vi "AssertControlDisable_Tests.vi"(11 "error in":errorcluster) -> (15 "error out":errorcluster)   [LabVIEW 2016, in "DronaTest.lvlib"]
uses:
  DronaTest.lvlib
  APIs/Stimulus/ControlValue/ValueSignalByPathString.vi
  APIs/Assert/AssertControlProperty/AssertControlDisable/AssertDisabled.vi
  APIs/Assert/AssertControlProperty/AssertControlDisable/AssertDisabledAndGrayedOut.vi
  APIs/Assert/AssertControlProperty/AssertControlDisable/AssertEnabled.vi
  <vilib>/addons/_JKI Toolkits/Caraya/classes/Test/Test.lvclass
  Drona.lvlib
  APIs/Stimulus/ControlValue/ControlValue.lvlib
  <vilib>/addons/_JKI Toolkits/Caraya/classes/Assert/Assert.lvclass
  APIs/Assert/AssertControlProperty/AssertControlDisable/AssertControlDisable.lvlib
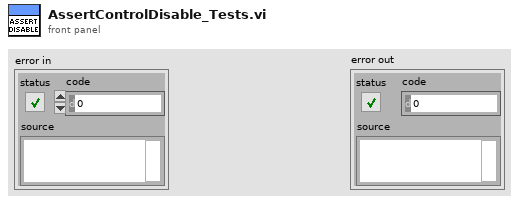
[diagram p1: front panel]
types:
  T1 = enum8{"Enabled", "Disabled", "Disabled and Grayed Out"}
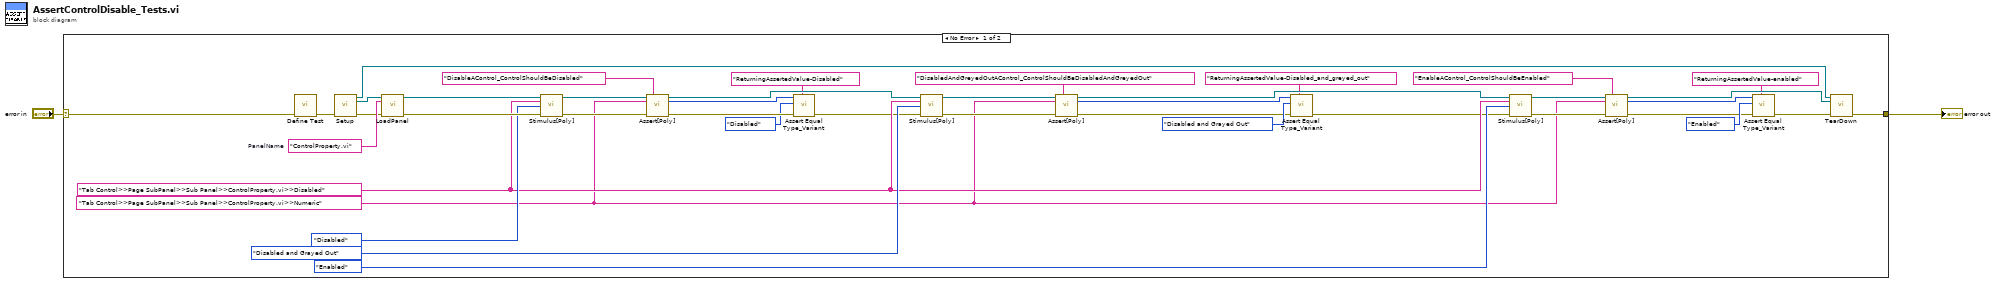
[diagram p0: block diagram]
diagram:
  n1 = case shown="No Error" "error in" {
    selector: "error in" -> [w43 w44]
    tunnel: [w20 w44] -> w1
    frame No Error {
      w24 = "Tab Control>>Page SubPanel>>Sub Panel>>ControlProperty.vi>>Numeric" ("Control Path")
      w25 = "Tab Control>>Page SubPanel>>Sub Panel>>ControlProperty.vi>>Disabled" ("Control Path")
      w42 = "ControlProperty.vi"  # PanelName
      n2 = call <vilib>:"Define Test.vi"("error in (no error)"=w43) -> ("error out"=w21:errorcluster)  [unwired: 9 in, 1 out]
      n3 = call "Setup.vi"("error in"=w21) -> ("Application Ref"=w18:refnum<vi>, "VI out"=w22:refnum<vi>, "error out"=w23:errorcluster)  [unwired: 12 in]
      n4 = call "LoadPanel.vi"("VI in"=w22, "Item Name"=w42, "error in"=w23) -> ("VI out"=w40:refnum<vi>, "error out"=w37:errorcluster)  [unwired: 11 in]
      n5 = call-poly "Stimulus[Poly].vi"("VI Reference In"=w40, "Control Path"=w25, "Value (Signaling)"=T1."Disabled" ("Disabled"), "error in"=w37) -> ("VI Reference Out"=w39:refnum<vi>, "error out"=w41:errorcluster)  [unwired: 10 in]
      n6 = call-poly "Assert[Poly].vi"("VI Reference In"=w39, "Test Label"="DisableAControl_ControlShouldBeDisabled" ("string"), "Control Path"=w24, "Error In"=w41) -> ("VI Reference Out"=w31:refnum<vi>, "Asserted Value"=w15:T1, "Error Out"=w17:errorcluster)  [unwired: 9 in]
      n7 = call <vilib>:"Assert Equal Type_Variant.vi"("Label"="ReturningAssertedValue-Disabled", "error in (no error)"=w17, "Y"=T1."Disabled" ("Asserted Value"), "X"=w15) -> ("error out"=w16:errorcluster)  [unwired: 6 in, 1 out]
      n8 = call-poly "Stimulus[Poly].vi"("VI Reference In"=w31, "Control Path"=w25, "Value (Signaling)"=T1."Disabled and Grayed Out" ("Disabled"), "error in"=w16) -> ("VI Reference Out"=w33:refnum<vi>, "error out"=w32:errorcluster)  [unwired: 10 in]
      n9 = call-poly "Assert[Poly].vi"("VI Reference In"=w33, "Test Label"="DisabledAndGreyedOutAControl_ControlShouldBeDisabledAndGreyedOut" ("string"), "Control Path"=w24, "Error In"=w32) -> ("VI Reference Out"=w27:refnum<vi>, "Asserted Value"=w8:T1, "Error Out"=w10:errorcluster)  [unwired: 9 in]
      n10 = call <vilib>:"Assert Equal Type_Variant.vi"("Label"="ReturningAssertedValue-Disabled_and_greyed_out", "error in (no error)"=w10, "Y"=T1."Disabled and Grayed Out" ("Asserted Value"), "X"=w8) -> ("error out"=w9:errorcluster)  [unwired: 6 in, 1 out]
      n11 = call-poly "Stimulus[Poly].vi"("VI Reference In"=w27, "Control Path"=w25, "Value (Signaling)"=T1."Enabled" ("Disabled"), "error in"=w9) -> ("VI Reference Out"=w29:refnum<vi>, "error out"=w30:errorcluster)  [unwired: 10 in]
      n12 = call-poly "Assert[Poly].vi"("VI Reference In"=w29, "Test Label"="EnableAControl_ControlShouldBeEnabled" ("string"), "Control Path"=w24, "Error In"=w30) -> ("VI Reference Out"=w19:refnum<vi>, "Asserted Value"=w3:T1, "Error Out"=w5:errorcluster)  [unwired: 9 in]
      n13 = call <vilib>:"Assert Equal Type_Variant.vi"("Label"="ReturningAssertedValue-enabled", "error in (no error)"=w5, "Y"=T1."Enabled" ("Asserted Value"), "X"=w3) -> ("error out"=w4:errorcluster)  [unwired: 6 in, 1 out]
      n14 = call "TearDown.vi"("Application Ref"=w18, "VI in"=w19, "error in (no error)"=w4) -> ("error out"=w20:errorcluster)  [unwired: 12 in]
    }
    frame Error {
    }
  }
  "error out" <- w1
